vi "Koheras_Seed_Laser_Power.vi"(7 "New Power":i8, 8 "Answer Length In":i32[](array[numeric]), 9 "Command In":string[](array[string]), 10 "Setted Seed Laser Power":i8, 11 "Modus In":i32) -> (0 "Answer Length Out":i32[](array[numeric]), 1 "Command Out":string[](array[string]), 3 "Modus Out":i32)   [LabVIEW 2009]
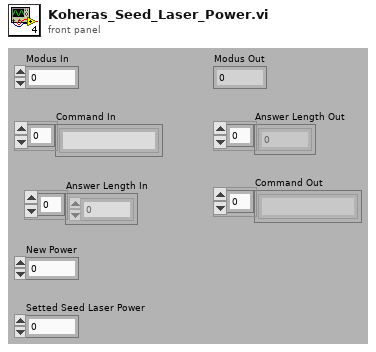
[diagram p1: front panel]
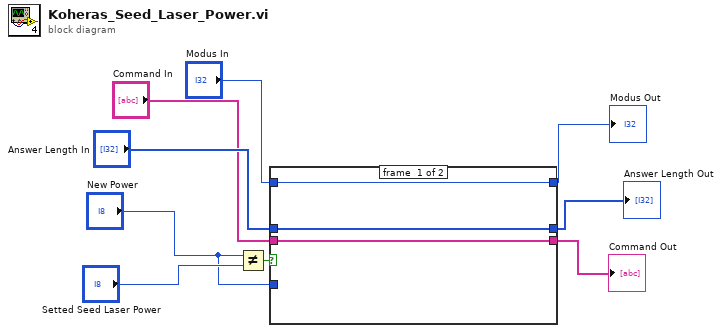
[diagram p0: block diagram]
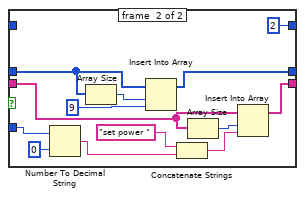
[diagram p2: hidden frame]
diagram:
  n1 = Not Equal?(x="New Power", y="Setted Seed Laser Power") -> (x != y?=w2:bool)
  n2 = case shown="True" w2 {
    tunnel: "Command In" -> [w11 w20]
    tunnel: "Answer Length In" -> [w12 w24]
    tunnel: [w12 w22] -> w5
    tunnel: [w11 w19] -> w6
    tunnel: "New Power" -> [_ w16]
    tunnel: "Modus In" -> [w10 _]
    tunnel: [w10 2 ("Modus Out")] -> w9
    frame #0 {
    }
    frame #1 {
      n3 = Number To Decimal String(number=w16, width (-)=i16 0) -> (decimal integer string=w15:string)
      n4 = Array Size(array=w24) -> (size(s)=w25:i32)
      n5 = Insert Into Array(array=w24, index=w25, new element=9 ("new element/subarray")) -> (w22:i32[])
      n6 = Concatenate Strings("set power " ("string"), w15) -> (w18:string)
      n7 = Array Size(array=w20) -> (size(s)=w21:i32)
      n8 = Insert Into Array(array=w20, index=w21, new element=w18) -> (w19:string[])
    }
  }
  "Modus Out" <- w9
  "Command Out" <- w6
  "Answer Length Out" <- w5
